vi "Actor Core.vi"(8 "error in":errorcluster, 11 "Measure Object in":refnum<class "Template Module.lvclass">) -> (0 "error out":errorcluster, 3 "Actor out":refnum<class "Actor.lvclass">)   [LabVIEW 2019, in "Template Module.lvclass"]
doc: "(<B>Filename</B>: Actor Framework.lvlib:Actor.lvclass:Actor Core.vi)\n\nReceives messages to the actor, reacts to them, and initiates any error handling that may shut the actor down.\n\nDescendant classes may override this VI to append parallel tasks for the actor to complete while it handles messages. Overrides use the Call Parent Method node."
uses:
  Template Module.lvclass
  C:/Program Files/National Instruments/LabVIEW 2019/vi.lib/ActorFramework/Actor/Actor.lvclass
  <vilib>/ActorFramework/Actor/Actor.lvclass
  Template Module.lvclass/Template Module.ctl
  <vilib>/ActorFramework/Actor/Actor.lvclass/Actor.ctl
  <vilib>/ActorFramework/Message Enqueuer/Message Enqueuer.lvclass/Message Enqueuer.ctl
  Template Module Messages/Open Item Msg/Open Item Msg.lvclass/Open Item Msg.ctl
  <vilib>/ActorFramework/Message Enqueuer/Init from Existing Queue.vi
  <vilib>/ActorFramework/Message Enqueuer/Enqueue.vi
  Template Module Messages/Open Item Msg/Open Item Msg.lvclass
  C:/Program Files/National Instruments/LabVIEW 2019/vi.lib/ActorFramework/Message/Message.lvclass
  <vilib>/ActorFramework/Message Priority Queue/Priority Enqueue.vi
  <vilib>/ActorFramework/Message Enqueuer/Message Enqueuer.lvclass
panel:
  in  "Configuration":cluster{"Placeholder":string}
  out "Name":string
  in  "No UI has been defined for this object":bool
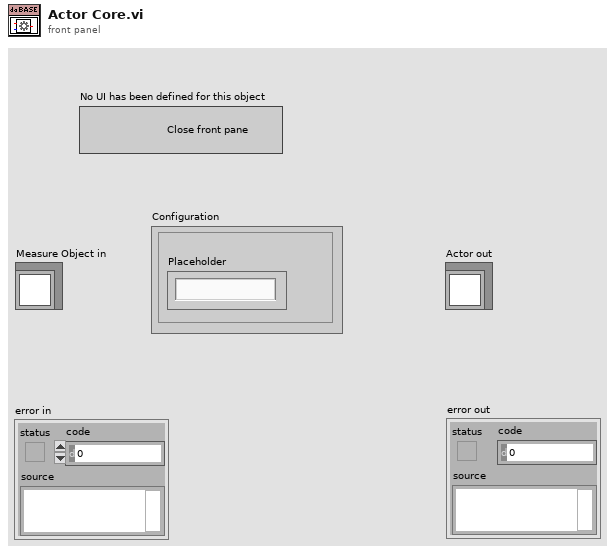
[diagram p1: front panel]
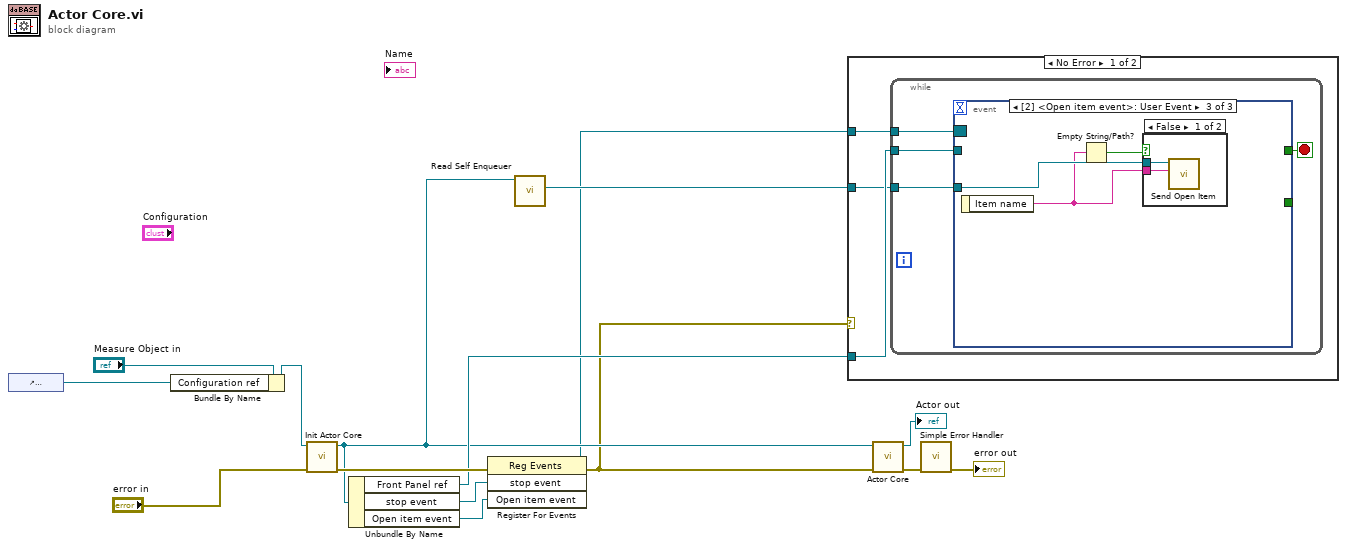
[diagram p0: block diagram]
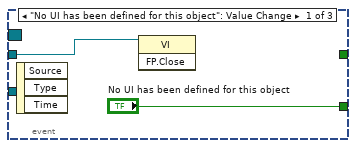
[diagram p2: hidden frame]
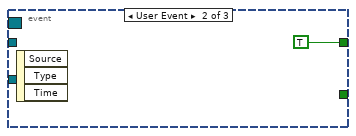
[diagram p3: hidden frame]
diagram:
  n1 = control-ref of="Configuration"() -> (w3:refnum<vi>)
  n2 = Bundle By Name(cluster="Measure Object in", "Configuration ref"=w3) -> (w4:refnum<class "Template Module.lvclass">)
  n3 = call-dynamic "Init Actor Core.vi"("error in (no error)"="error in", "Measure Object in"=w4) -> ("error out"=w11:errorcluster, "Measure Object out"=w8:refnum<class "Template Module.lvclass">)  [unwired: 8 in]
  n4 = Unbundle By Name(w8) -> ("Front Panel ref"=w9:refnum<vi>, "stop event"=w10:refnum<user-event>, "Open item event"=w5:refnum<user-event>)
  n5 = register-events(error in=w11, w10, w5) -> (reference out=w2:refnum<event-registration>, error out=w6:errorcluster)  [unwired: 1 in]
  n6 = call <vilib>:"Read Self Enqueuer.vi"("Actor"=w8) -> ("Self Enqueuer"=w7:refnum<class "Message Enqueuer.lvclass">)  [unwired: 10 in]
  n7 = case shown="No Error" w6 {
    tunnel: w9 -> [w18 _]
    tunnel: w2 -> [w17 _]
    tunnel: w7 -> [w16 _]
    frame No Error {
      n8 = while {
        tunnel: w18 -> [w22]
        tunnel: w17 -> [w21]
        tunnel: w16 -> [w19]
        stop <- w20 stop-if-true
        n9 = event shown="[2] <Open item event>: User Event" {
          selector: w21 -> [_ _ _]
          dyn-events: _ -> [_ _ _]
          timeout: _ -> [_ _ _]
          tunnel: w22 -> [w24 _ _]
          tunnel: ["No UI has been defined for this object" _ _] -> _
          tunnel: [_ TRUE _] -> w20
          tunnel: w19 -> [_ _ w28]
          event "No UI has been defined for this object": Value Change {
            n10 = event-data() -> ()  [unwired: 1 in, 3 out]
            n11 = invoke class="VI" method="FP.Close"(reference=w24) -> ()  [unwired: 2 in, 3 out]
          }
          event User Event {
            n12 = event-data() -> ()  [unwired: 1 in, 3 out]
          }
          event User Event {
            n13 = event-data() -> ("Item name"=w27:string)  [unwired: 1 in]
            n14 = Empty String/Path?(string/path=w27) -> (empty?=w26:bool)
            n15 = case shown="False" w26 {
              tunnel: w28 -> [w30 _]
              tunnel: w27 -> [w29 _]
              frame False {
                n16 = call "Send Open Item.vi"("Item name"=w29, "Message Enqueuer"=w30) -> ()  [unwired: 8 in, 2 out]
              }
              frame True {
              }
            }
          }
        }
      }
    }
    frame Error {
    }
  }
  n17 = call-parent "Actor Core.vi"("error in"=w6, "Actor in"=w8) -> ("error out"=w15:errorcluster, "Actor out"=→"Actor out":refnum<class "Actor.lvclass">)  [unwired: 8 in]
  n18 = call <vilib>:"Simple Error Handler.vi"("error in (no error)"=w15) -> ("error out"=→"error out":errorcluster)  [unwired: 4 in, 4 out]
